vi "HP 3458A Read Digital Sample Memory RJI.vi"(0 "VISA session":refnum<visa-resource-name>, 5 "First Read in Memory Location (0)":i32, 7 "Numbers of Samples (100)":i32=100, 9 "Output Format (0:ASCII)":T1(ring), 11 "error in (no error)":errorcluster) -> (4 "dup VISA session":refnum<visa-resource-name>, 8 "Output Array":dbl[](array[numeric]) format="%^.3e", 15 "error out":errorcluster)   [LabVIEW 2014, in "SamplerPlugins.lvlib" / "HP3458aDMM.lvclass"]
doc: "It reads in the data from the instrument's memory, in an ascending order from first memory location to last. After typecasting the data into ASCII format, it then outputs each value as an element in the array."
uses:
  HP3458aDMM.lvclass
  <instrlib>/Agilent 3458/Agilent 3458.lvlib
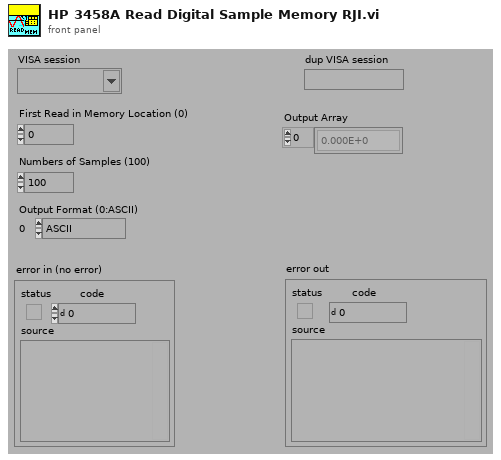
[diagram p1: front panel]
types:
  T1 = enum16{"ASCII", "Single Real", "Double Real", "Single Integer", "Double Integer"}
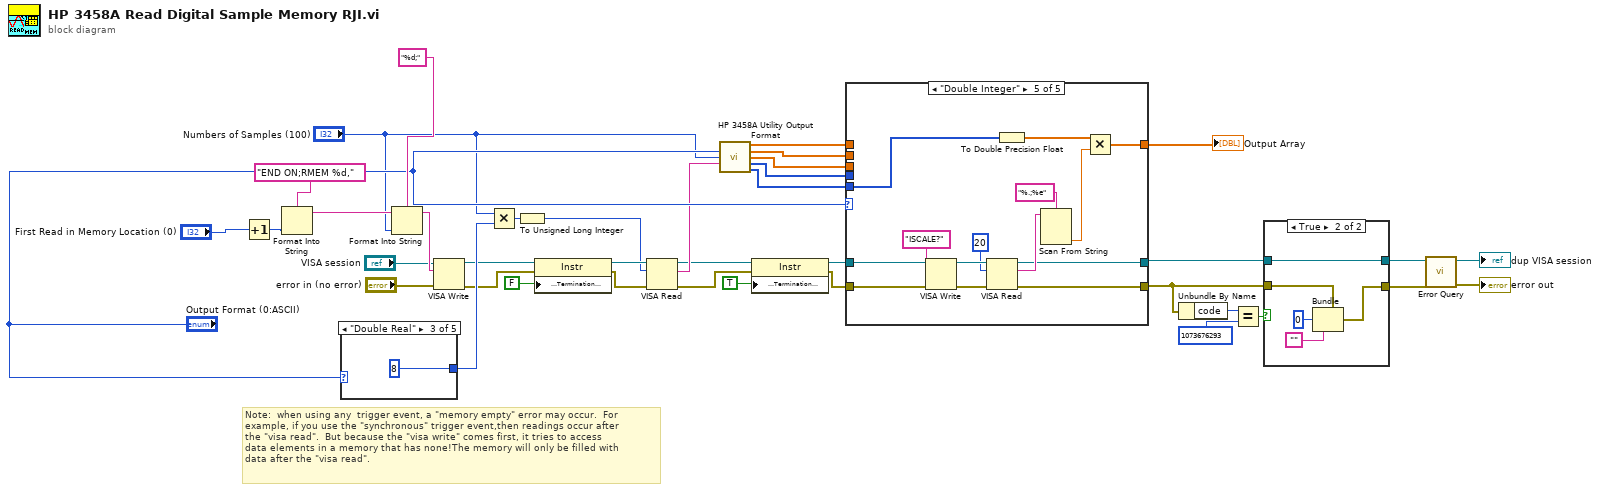
[diagram p0: block diagram]
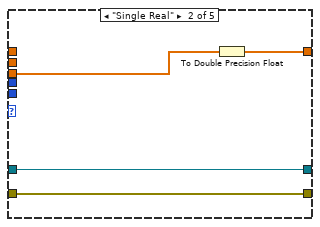
[diagram p4: hidden frame]
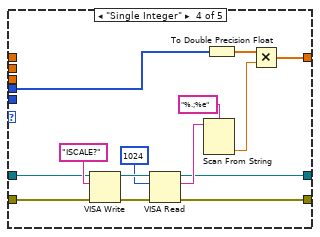
[diagram p6: hidden frame]
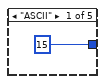
[diagram p7: hidden frame]
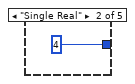
[diagram p8: hidden frame]
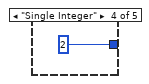
[diagram p9: hidden frame]
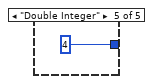
[diagram p10: hidden frame]
diagram:
  # "Note:  when using any  trigger event, a \"memory empty\" error may occur.  For \nexample, if you use the \"synchronous\" trigger event,then readings occur after \nthe \"visa read\".  But because the \"visa write\" comes first, it tries to access \ndata elements in a memory that has none!The memory will only be filled with \ndata after the \"visa read\"."
  n1 = Increment(x="First Read in Memory Location (0)") -> (x+1=w32:i32)
  n2 = Format Into String(format string="END ON;RMEM %d,", w32) -> (resulting string=w38:string)  [unwired: 2 in, 1 out]
  n3 = case shown="\"Double Real\"" "Output Format (0:ASCII)" {
    tunnel: [15 ("15 bytes per reading") 4 ("4 bytes per reading") 8 ("8 bytes per reading") 2 ("2 bytes per reading") 4 ("4 bytes per reaing")] -> w23
    frame "ASCII" {
    }
    frame "Single Real" {
    }
    frame "Double Real" {
    }
    frame "Single Integer" {
    }
    frame "Double Integer" {
    }
  }
  n4 = Format Into String(format string="%d;", initial string=w38, "Numbers of Samples (100)") -> (resulting string=w36:string)  [unwired: 1 in, 1 out]
  n5 = VISA Write(VISA resource name="VISA session", write buffer=w36, error in (no error)="error in (no error)") -> (VISA resource name out=w10:refnum<visa-resource-name>, error out=w2:errorcluster)  [unwired: 1 out]
  n6 = Multiply(x="Numbers of Samples (100)", y=w23) -> (x*y=w31:i32)
  n7 = To Unsigned Long Integer(number=w31) -> (unsigned 32bit integer=w1:u32)
  n8 = property class="Instr"(reference=w10, error in=w2, "Message Based Settings:Termination Character Enable"=FALSE ("TermChar En")) -> (reference out=w4:refnum<visa-resource-name>, error out=w3:errorcluster)
  n9 = VISA Read(VISA resource name=w4, byte count=w1, error in (no error)=w3) -> (VISA resource name out=w19:refnum<visa-resource-name>, read buffer=w28:string, error out=w18:errorcluster)  [unwired: 1 out]
  n10 = call "HP 3458A Utility Output Format.vi"("Output Format (0:ASCII)"="Output Format (0:ASCII)", "Numbers of Reading (1)"="Numbers of Samples (100)", "Input String"=w28) -> ("Output Data (ASCII)"=w26:dbl[], "Output Data (Double Real)"=w24:dbl[], "Output Data (Single Real)"=w25:sgl[], "Output Data (Single Integer)"=w30:i16[], "Output Data (Double Integer)"=w27:i32[])  [unwired: 8 in]
  n11 = property class="Instr"(reference=w19, error in=w18, "Message Based Settings:Termination Character Enable"=TRUE ("TermChar En")) -> (reference out=w16:refnum<visa-resource-name>, error out=w17:errorcluster)
  n12 = case shown="\"Double Integer\"" "Output Format (0:ASCII)" {
    tunnel: w30 -> [_ _ _ w59 _]
    tunnel: [w47 w48 w54 w58 w72] -> w22
    tunnel: [w46 w50 w53 w62 w76] -> w12
    tunnel: [w45 w49 w52 w61 w75] -> w11
    tunnel: w27 -> [_ _ _ _ w74]
    tunnel: w26 -> [w47 _ _ _ _]
    tunnel: w25 -> [_ w51 _ _ _]
    tunnel: w24 -> [_ _ w54 _ _]
    tunnel: w16 -> [w46 w50 w53 w56 w70]
    tunnel: w17 -> [w45 w49 w52 w55 w69]
    frame "ASCII" {
    }
    frame "Single Real" {
      n13 = To Double Precision Float(number=w51) -> (double precision float=w48:dbl[])
    }
    frame "Double Real" {
    }
    frame "Single Integer" {
      n14 = VISA Write(VISA resource name=w56, write buffer="ISCALE?" ("write buffer (\"\")"), error in (no error)=w55) -> (VISA resource name out=w67:refnum<visa-resource-name>, error out=w66:errorcluster)  [unwired: 1 out]
      n15 = VISA Read(VISA resource name=w67, byte count=u32 1024 ("byte count (0)"), error in (no error)=w66) -> (VISA resource name out=w62:refnum<visa-resource-name>, read buffer=w64:string, error out=w61:errorcluster)  [unwired: 1 out]
      n16 = Scan From String(format string="%.;%e", input string=w64) -> (output 1=w60:dbl)  [unwired: 3 in, 3 out]
      n17 = To Double Precision Float(number=w59) -> (double precision float=w57:dbl[])
      n18 = Multiply(x=w57, y=w60) -> (x*y=w58:dbl[])
    }
    frame "Double Integer" {
      n19 = VISA Write(VISA resource name=w70, write buffer="ISCALE?" ("write buffer (\"\")"), error in (no error)=w69) -> (VISA resource name out=w81:refnum<visa-resource-name>, error out=w80:errorcluster)  [unwired: 1 out]
      n20 = VISA Read(VISA resource name=w81, byte count=u32 20 ("byte count (0)"), error in (no error)=w80) -> (VISA resource name out=w76:refnum<visa-resource-name>, read buffer=w78:string, error out=w75:errorcluster)  [unwired: 1 out]
      n21 = To Double Precision Float(number=w74) -> (double precision float=w71:dbl[])
      n22 = Scan From String(format string="%.;%e", input string=w78) -> (output 1=w73:dbl)  [unwired: 3 in, 3 out]
      n23 = Multiply(x=w71, y=w73) -> (x*y=w72:dbl[])
    }
  }
  "Output Array" <- w22
  n24 = Unbundle By Name(w11) -> ("code"=w15:i32)
  n25 = Equal?(x=w15, y=1073676293 ("The specified termination character  was read")) -> (x = y?=w13:bool)
  n26 = case shown="True" w13 {
    tunnel: w11 -> [w84 w89]
    tunnel: [w84 w88] -> w7
    tunnel: [w83 w85] -> w8
    tunnel: w12 -> [w83 w85]
    frame False {
    }
    frame True {
      n27 = Bundle(cluster=w89, "code"=0, "source"="" ("Empty String")) -> (w88:errorcluster)  [unwired: 1 in]
    }
  }
  n28 = call <instrlib>:"Error Query.vi"("error in (no error)"=w7, "VISA resource name"=w8) -> ("error out"=→"error out":errorcluster, "VISA resource name out"=→"dup VISA session":refnum<visa-resource-name>)  [unwired: 6 in, 2 out]
